vi "Handle Command.vi"(8 "error in":errorcluster, 10 "Reset Red Laser Rep Rate in":refnum<class "Reset Red Laser Rep Rate.lvclass">, 11 "Object In":refnum<class>) -> (0 "error out":errorcluster, 1 "Command Successful?":bool, 2 "Reset Red Laser Rep Rate out":refnum<class "Reset Red Laser Rep Rate.lvclass">, 3 "Object Out":refnum<class>)   [LabVIEW 2014, in "eCRDS Library.lvlib" / "Reset Red Laser Rep Rate.lvclass"]
doc: "Abstract method for accomplishing the execution of a command directed to an instrument object on the wire."
uses:
  Reset Red Laser Rep Rate.lvclass
  Main/eCRDS.lvclass
  Main/eCRDS.lvclass/eCRDS.ctl
  reusable/Instrument/Instrument.lvclass/Instrument.ctl
  Reset Red Laser Rep Rate.lvclass/Reset Red Laser Rep Rate.ctl
  Main/Accessors/Read Red DAQ.vi
  Main/Accessors/Read Red Tasks.vi
  Main/Accessors/Read Blue Tasks.vi
  reusable/Instrument/Read Log Session.vi
  Main/Accessors/Write Red DAQ.vi
  <vilib>/DAQmx/configure/timing.llb/DAQmx Timing (Implicit).vi
  <userlib>/_Session Fwk/Session - Root.lvclass
  <resource>/objmgr/daqmx.rc
  reusable/Session APIs/Session Log/System Log.lvclass
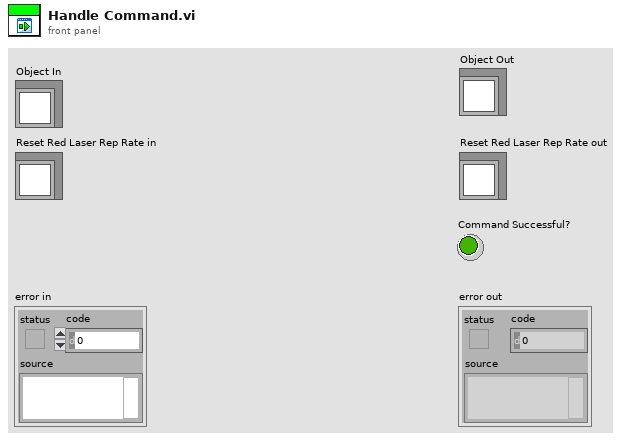
[diagram p1: front panel]
types:
  T1 = cluster{"Rate (MHz)":dbl, "Laser Rep (Hz)":dbl, "Laser DC (%)":dbl}
  T2 = cluster{"CLk":refnum<k21>, "AI":refnum<k21>, "DO":refnum<k21>}
  T3 = typedef "Session - Root.lvclass/Session Handle.ctl" = refnum<data-value>
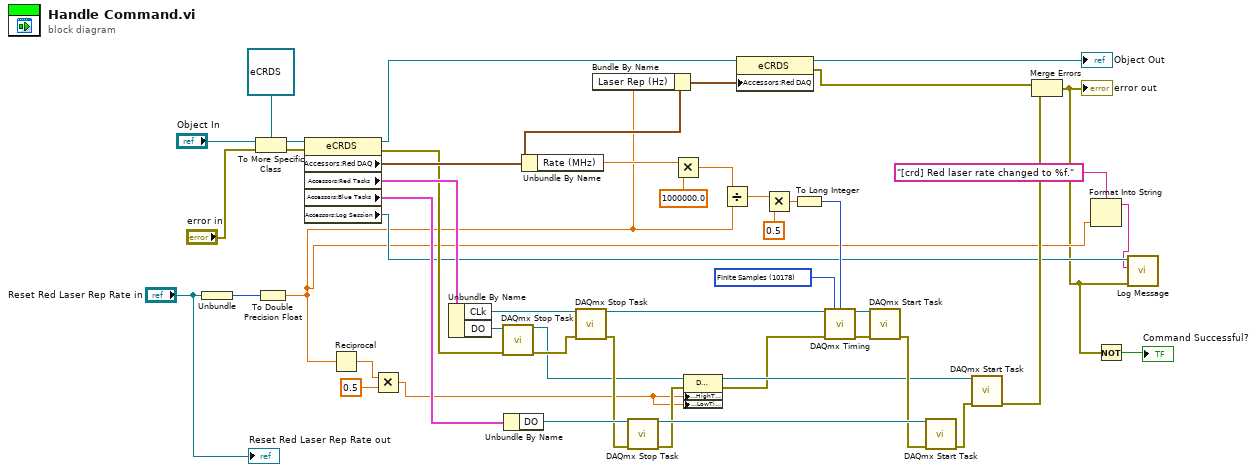
[diagram p0: block diagram]
diagram:
  w36 = 10178 items=["Finite Samples"=10178, "Continuous Samples"=10123, "Hardware Timed Single Point"=12522] ("sample mode")
  n1 = Unbundle("Reset Red Laser Rep Rate in") -> (w43:i32)
  n2 = To More Specific Class(target class=refnum<class "eCRDS.lvclass"> refnum ("eCRDS"), reference="Object In", error in="error in") -> (specific class reference=w45:refnum<class "eCRDS.lvclass">, error out=w42:errorcluster)
  n3 = To Double Precision Float(number=w43) -> (double precision float=w5:dbl)
  n4 = property class="eCRDS"(reference=w45, error in=w42) -> (reference out=w21:refnum<class "eCRDS.lvclass">, error out=w24:errorcluster, "Accessors:Red DAQ"=w44:T1, "Accessors:Red Tasks"=w41:T2, "Accessors:Blue Tasks"=w40:T2, "Accessors:Log Session"=w7:T3)
  n5 = Reciprocal(x=w5) -> (1/x=w10:dbl)
  n6 = Multiply(x=w10, y=0.5) -> (x*y=w8:dbl)
  n7 = Unbundle By Name(w41) -> ("CLk"=w37:refnum<k21>, "DO"=w39:refnum<k21>)
  n8 = call <vilib>:"DAQmx Stop Task.vi"("task/channels in"=w39, "error in"=w24) -> ("task out"=w14:refnum<k21>, "error out"=w23:errorcluster)  [unwired: 12 in]
  n9 = Unbundle By Name(w40) -> ("DO"=w38:refnum<k21>)
  n10 = Unbundle By Name(w44) -> ("Rate (MHz)"=w34:dbl)
  n11 = call <vilib>:"DAQmx Stop Task.vi"("task/channels in"=w37, "error in"=w23) -> ("task out"=w35:refnum<k21>, "error out"=w22:errorcluster)  [unwired: 12 in]
  n12 = Bundle By Name(cluster=w44, "Laser Rep (Hz)"=w5) -> (w20:T1)
  n13 = call <vilib>:"DAQmx Stop Task.vi"("task/channels in"=w38, "error in"=w22) -> ("task out"=w25:refnum<k21>, "error out"=w11:errorcluster)  [unwired: 12 in]
  n14 = Multiply(x=w34, y=1000000.0) -> (x*y=w32:dbl)
  n15 = property class="DAQmx Channel"(reference=w14, error in=w11, "CO.Pulse.HighTime"=w8, "CO.Pulse.LowTime"=w8) -> (reference out=w13:refnum<k21>, error out=w12:errorcluster)
  n16 = Divide(x=w32, y=w5) -> (x/y=w31:dbl)
  n17 = property class="eCRDS"(reference=w21, "Accessors:Red DAQ"=w20) -> (reference out=→"Object Out":refnum<class "eCRDS.lvclass">, error out=w19:errorcluster)  [unwired: 1 in]
  n18 = Multiply(x=w31, y=0.5) -> (x*y=w29:dbl)
  n19 = To Long Integer(number=w29) -> (32bit integer=w28:i32)
  n20 = call-poly <vilib>:"DAQmx Timing.vi"("task/channels in"=w35, "sample mode"=w36, "samples per channel"=w28, "error in"=w12) -> ("task out"=w27:refnum<k21>, "error out"=w26:errorcluster)  [unwired: 10 in]
  n21 = call <vilib>:"DAQmx Start Task.vi"("task/channels in"=w27, "error in"=w26) -> ("error out"=w17:errorcluster)  [unwired: 12 in, 1 out]
  n22 = call <vilib>:"DAQmx Start Task.vi"("task/channels in"=w25, "error in"=w17) -> ("error out"=w16:errorcluster)  [unwired: 12 in, 1 out]
  n23 = call <vilib>:"DAQmx Start Task.vi"("task/channels in"=w13, "error in"=w16) -> ("error out"=w15:errorcluster)  [unwired: 12 in, 1 out]
  n24 = Merge Errors(w19, w15) -> (w3:errorcluster)
  "error out" <- w3
  n25 = Format Into String(format string="[crd] Red laser rate changed to %f.", w5) -> (resulting string=w4:string)  [unwired: 2 in, 1 out]
  n26 = Not(x=w3) -> (.not. x?=→"Command Successful?":bool)
  n27 = call "Log Message.vi"("error in"=w3, "MSG In"=w4, "session in"=w7) -> ()  [unwired: 7 in, 2 out]
  "Reset Red Laser Rep Rate out" <- "Reset Red Laser Rep Rate in"
